vi "Simple Drive.vi"() -> ()   [LabVIEW 2013]
uses:
  <vilib>/Platform/TimedLoop/XDataNode/timing_clust.ctl
  <vilib>/Platform/TimedLoop/XDataNode/nitl_modes.ctl
  <vilib>/Platform/TimedLoop/XDataNode/wakeup.ctl
  <vilib>/Rock Robotics/WPI/SafetyOutput/WPI_SafetyOutputConfigMenu.ctl
  <vilib>/Rock Robotics/WPI/Joystick/WPI_JoystickDeviceEnum.ctl
  <vilib>/Rock Robotics/SystemInterfaces/DIO/FPGA_DIOPWMChannel.ctl
  Program Files (x86)/National Instruments/LabVIEW 2013/examples/FRC/I2C/ADXL345 I2C/Driver/ADXL345 I2C Range.ctl
  <vilib>/Rock Robotics/SystemInterfaces/Typedef/FPGA_TypedefDigitalModule.ctl
  Program Files (x86)/National Instruments/LabVIEW 2013/examples/FRC/I2C/ADXL345 I2C/Driver/ADXL345 I2C Axis.ctl
  <vilib>/Rock Robotics/WPI/RobotDrive/WPI_RobotDriveOpen2MotorWithJaguar.vi
  <vilib>/Rock Robotics/WPI/RobotDrive/WPI_RobotDriveArcadeDrive_Standard(NoSaturation).vi
  <vilib>/Platform/TimedLoop/XDataNode/XDataNode.xnode
  <vilib>/Platform/TimedLoop/XDataNode/XDNodeRunTimeDep.lvlib
panel:
  out "Acceleration":dbl
  out "Battery Voltage":dbl
  in  "Joystick enbled":bool=TRUE
  in  "Left axis":dbl(slide) step=0.1 scale=-1.0..1.0
  in  "Right axis":dbl(slide) step=0.1 scale=-1.0..1.0
  in  "stop":bool
  # "Drive Motors"
  # "Encoder"
  # "Motion"
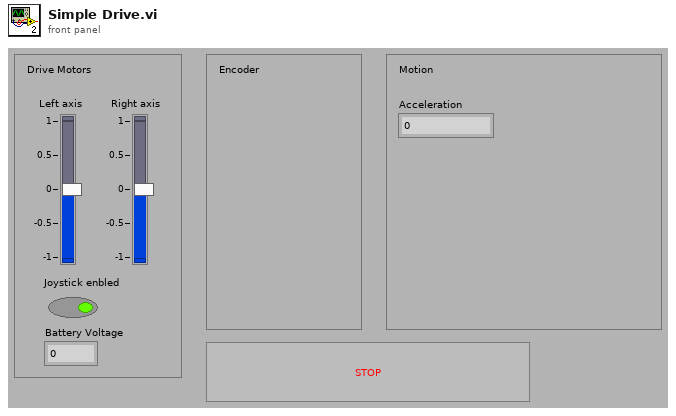
[diagram p1: front panel]
types:
  T1 = typedef "FPGA_TypedefDigitalModule.ctl" = enum16{"Digital Module 1", "Digital Module 2"}
  T2 = typedef "ADXL345 I2C Range.ctl" = u8
  T3 = typedef "FPGA_DIOPWMChannel.ctl" = enum8{"PWM 1", "PWM 2", "PWM 3", "PWM 4", "PWM 5", "PWM 6", "PWM 7", "PWM 8", "PWM 9", "PWM 10", "Invalid"}
  T4 = typedef "WPI_JoystickDeviceEnum.ctl" = enum16{"USB 1", "USB 2", "USB 3", "USB 4", "Kinect 1", "Kinect 2"}
  T5 = typedef "WPI_SafetyOutputConfigMenu.ctl" = enum16{"Enable", "Disable"}
  T6 = typedef "WPI_RobotDriveDevRef.ctl" = cluster{"DevStatus":errorcluster, "Motors[]":T7[], "Square Inputs":bool, "Max Output":dbl, "Isochronous":bool}
  T7 = typedef "WPI_MotorControlDeviceRef.ctl" = cluster{"DeviceStatus":errorcluster, "Type":enum16{"PWM", "CAN"}, "PWM":cluster{"Digital Module":T1, "PWM Channel":T3, "DeadBand":T8}, "CAN":cluster{"Device Number":u8, "Control Mode":T9, "Semaphore":T10, "Max Vout":dbl}, "Invert":bool, "TransformRef":T11, "InvTransformRef":T11}
  T8 = typedef "WPI_PWMDeadband.ctl" = cluster{"Name":string, "maxPositivePwm":i32, "minPositivePwm":i32, "centerPwm":i32, "maxNegativePwm":i32, "minNegativePwm":i32, "angularRange":u16}
  T9 = typedef "WPI_CANJaguar_ControlMode.ctl" = enum8{"Percent VBus", "Current", "Speed", "Position", "Voltage"}
  T10 = typedef "Semaphore RefNum" = refnum<k1>
  T11 = typedef "WPI_PWMTransform_ConPane.ctl" = refnum<vi>
  T12 = typedef "WPI_I2CDevRef.ctl" = cluster{"DevStatus":errorcluster, "Digital Module":T1, "Device Address":u8}
  T13 = typedef "XDNodeRunTimeDep.lvlib/timing_clust.ctl" = cluster{"Expected End [f-1]":u64, "Actual End [f-1]":u64, "Finished Late? [f-1]":bool, "Expected End [i-1]":u64, "Actual End [i-1]":u64, "Finished Late? [i-1]":bool, "Expected Start [i]":u64, "Actual Start [i]":u64, "Expected Start [f]":u64, "Actual Start [f]":u64, "Source Name":string, "Structure Name":string, "Period":i64, "Deadline":i64, "Offset":i64, "Start":i64, "Priority":i32, "Timeout":i32, "Mode":T14, "Wakeup Reason":T15, "Error":errorcluster, "Source Type":string, "Secondary Source Type":string, "Global End Time":u64, "Global Start Time":u64, "Frame Duration":u64, "Iteration Duration":u64, "Assigned CPU":i32, "I/O Scan Engine Mode":u32}
  T14 = typedef "XDNodeRunTimeDep.lvlib/nitl_modes.ctl" = enum32{"No Change", "Process missed periods, maintain original phase", "Discard missed periods, maintain original phase", "Process missed periods, ignore original phase", "Discard missed periods, ignore original phase"}
  T15 = typedef "XDNodeRunTimeDep.lvlib/wakeup.ctl" = enum32{"Normal", "Aborted", "Asynchronous wakeup", "Timing source error", "Timed loop error", "Timeout"}
  T16 = typedef "WPI_JoystickDevRef.ctl" = cluster{"Device":T4}
  T17 = typedef "ADXL345 I2C Axis.ctl" = u8
  T18 = cluster{"axis 1 (x)":dbl, "axis 2 (y)":dbl, "axis 3 (throttle)":dbl, "axis 4":dbl, "axis 5":dbl, "axis 6":dbl}
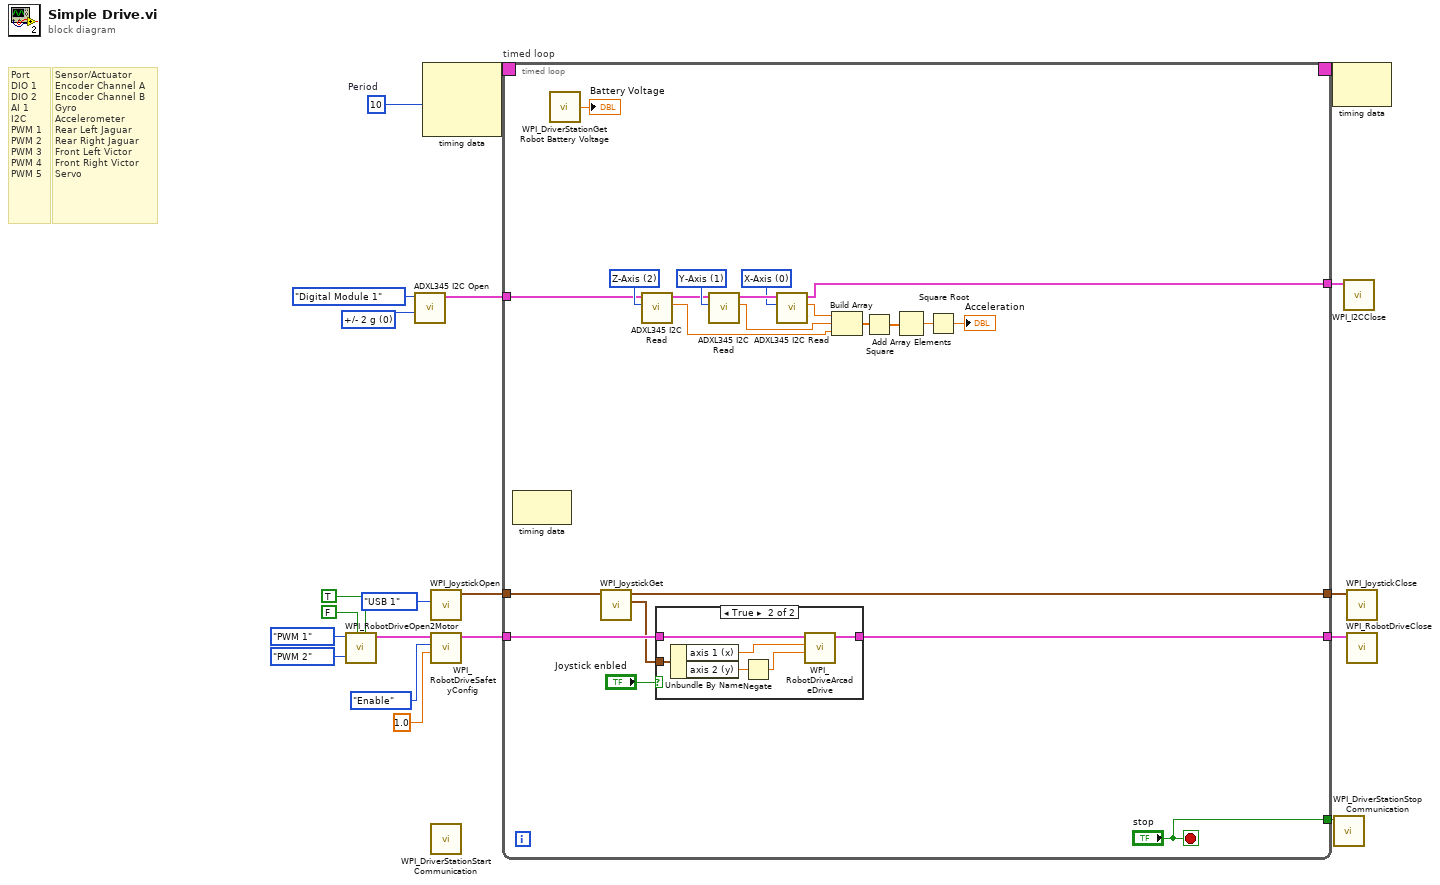
[diagram p0: block diagram]
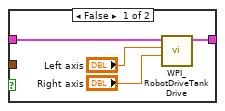
[diagram p2: hidden frame]
diagram:
  w4 = T2 0 items=["+/- 2 g", "+/- 4 g", "+/- 8 g", "+/- 16 g"] ("Range")
  w18 = i64 10  # Period
  # "Sensor/Actuator\nEncoder Channel A\nEncoder Channel B\nGyro\nAccelerometer\nRear Left Jaguar\nRear Right Jaguar\nFront Left Victor\nFront Right Victor\nServo"
  # "Port\nDIO 1\nDIO 2\nAI 1\nI2C\nPWM 1\nPWM 2\nPWM 3\nPWM 4\nPWM 5"
  n1 = call-poly <vilib>:"WPI_RobotDriveOpen2Motor.vi"("Right Motor Inverted"=TRUE, "Left Motor Inverted"=FALSE, "Right Motor"=FPGA_DIOPWMChannel."PWM 2", "Left Motor"=FPGA_DIOPWMChannel."PWM 1") -> ("RobotDriveDevRef"=w17:T6)  [unwired: 6 in, 1 out]
  n2 = call "ADXL345 I2C Open.vi"("Range"=w4, "DIO Module (Module 1)"=FPGA_TypedefDigitalModule."Digital Module 1") -> ("I2CDevRef"=w3:T12)  [unwired: 2 in, 7 out]
  n3 = node-c288(w18) -> (w20:T13)  [unwired: 2 out]
  n4 = call <vilib>:"WPI_JoystickOpen.vi"("JoystickDevice"=WPI_JoystickDeviceEnum."USB 1") -> ("JoystickDevRef"=w13:T16)  [unwired: 10 in]
  n5 = call <vilib>:"WPI_RobotDriveSafetyConfig.vi"("timeout (s)"=1.0, "mode"=WPI_SafetyOutputConfigMenu."Enable", "RobotDriveDevRef"=w17) -> ("RobotDriveDevRef"=w16:T6)  [unwired: 7 in, 1 out]
  n6 = call <vilib>:"WPI_DriverStationStart Communication.vi"() -> ()  [unwired: 1 in, 11 out]
  n7 = timed-loop "timed loop" {
    timing: w20 -> [_]
    timing-out: [_] -> w19
    tunnel: w16 -> [w41]
    tunnel: [w36] -> w14
    tunnel: w13 -> [w42]
    tunnel: [w37] -> w10
    tunnel: ["stop"] -> w5
    tunnel: w3 -> [w23]
    tunnel: [w22] -> w2
    stop <- "stop" stop-if-true
    w31 = T17 2 items=["X-Axis", "Y-Axis", "Z-Axis"] ("Axis")
    w33 = T17 0 items=["X-Axis", "Y-Axis", "Z-Axis"] ("Axis")
    w32 = T17 1 items=["X-Axis", "Y-Axis", "Z-Axis"] ("Axis")
    n8 = node-c288() -> ()  [unwired: 2 out]
    n9 = call <vilib>:"WPI_DriverStationGet Robot Battery Voltage.vi"() -> ("robot battery voltage"=→"Battery Voltage":dbl)  [unwired: 14 in, 1 out]
    n10 = call <vilib>:"WPI_JoystickGet.vi"("JoystickDevRef"=w42) -> ("Axes"=w40:T18, "JoystickDevRef"=w37:T16)  [unwired: 4 in, 1 out]
    n11 = call "ADXL345 I2C Read.vi"("Axis"=w31, "I2CDevRef"=w23) -> ("Acceleration"=w21:dbl, "I2CDevRef Out"=w30:T12)  [unwired: 1 in, 7 out]
    n12 = case shown="True" "Joystick enbled" {
      tunnel: w41 -> [w46 w49]
      tunnel: [w47 w48] -> w36
      tunnel: w40 -> [_ w53]
      frame False {
        n13 = call <vilib>:"WPI_RobotDriveTankDrive.vi"("Right axis value"="Right axis", "Left axis value"="Left axis", "RobotDriveDevRef"=w46) -> ("RobotDriveDevRef"=w47:T6)  [unwired: 6 in, 2 out]
      }
      frame True {
        n14 = Unbundle By Name(w53) -> ("axis 1 (x)"=w52:dbl, "axis 2 (y)"=w51:dbl)
        n15 = Negate(x=w51) -> (-x=w50:dbl)
        n16 = call-poly <vilib>:"WPI_RobotDriveArcadeDrive.vi"("Y axis value"=w50, "X axis value"=w52, "RobotDriveDevRef"=w49) -> ("RobotDriveDevRef"=w48:T6)  [unwired: 6 in, 2 out]
      }
    }
    n17 = call "ADXL345 I2C Read.vi"("Axis"=w32, "I2CDevRef"=w30) -> ("Acceleration"=w24:dbl, "I2CDevRef Out"=w34:T12)  [unwired: 1 in, 7 out]
    n18 = call "ADXL345 I2C Read.vi"("Axis"=w33, "I2CDevRef"=w34) -> ("Acceleration"=w29:dbl, "I2CDevRef Out"=w22:T12)  [unwired: 1 in, 7 out]
    n19 = Build Array(w29, w24, w21) -> (w28:dbl[])
    n20 = Square(x=w28) -> (x^2=w27:dbl[])
    n21 = Add Array Elements(numeric array=w27) -> (sum=w26:dbl)
    n22 = Square Root(x=w26) -> (sqrt(x)=→"Acceleration":dbl)
  }
  n23 = node-c288(w19) -> ()  [unwired: 1 out]
  n24 = call <vilib>:"WPI_DriverStationStop Communication.vi"("StopCommunication"=w5) -> ()  [unwired: 10 in, 1 out]
  n25 = call <vilib>:"WPI_I2CClose.vi"("I2CDevRef"=w2) -> ()  [unwired: 10 in, 1 out]
  n26 = call <vilib>:"WPI_JoystickClose.vi"("JoystickDevRef"=w10) -> ()  [unwired: 11 in]
  n27 = call <vilib>:"WPI_RobotDriveClose.vi"("RobotDriveDevRef"=w14) -> ()  [unwired: 10 in, 1 out]
